vi "SortArrayData.vi"(4 "Stacked Data":i16[][][][](array[numeric]), 6 "Atts":dbl[][](array[numeric])) -> (0 "Syth App Data":i16[][][](array[numeric]), 1 "Number of Planes":i32, 2 "Att (dB)":sgl[](array[numeric]))   [LabVIEW 2022 SP3]
panel:
  in  "Case Constant\n(See Context Help)":bool=TRUE
  out "size(s) 2":i32[](array[numeric])
  out "size(s)":i32[](array[numeric])
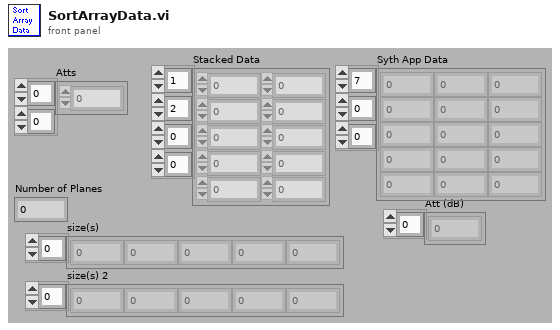
[diagram p1: front panel]
types:
  T1 = cluster{"[0]":i32, "[1]":i32, "[2]":i32, "[3]":i32}
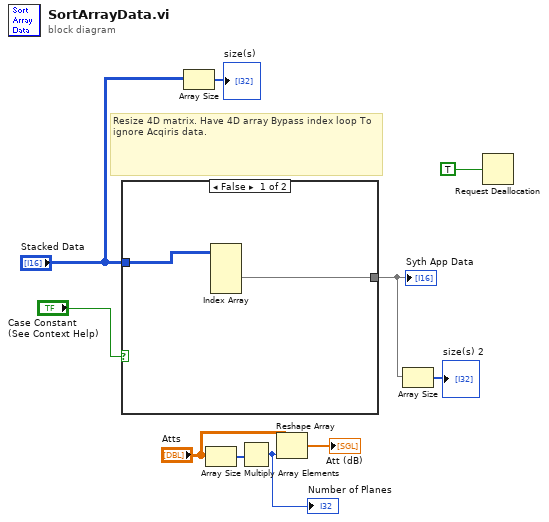
[diagram p0: block diagram]
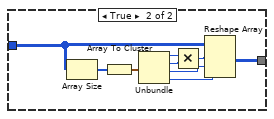
[diagram p2: hidden frame]
diagram:
  # "Resize 4D matrix. Have 4D array Bypass index loop To ignore Acqiris data."
  n1 = case shown="False" "Case Constant\n(See Context Help)" {
    tunnel: "Stacked Data" -> [w11 w13]
    tunnel: [w12 w14] -> w5
    frame False {
      n2 = Index Array(array=w11) -> (element=w12:i16[][][])  [unwired: 4 in]
    }
    frame True {
      n3 = Array Size(array=w13) -> (size(s)=w16:i32[])
      n4 = Array To Cluster(array=w16) -> (cluster=w17:T1)
      n5 = Unbundle(w17) -> ("[0]"=w15:i32, "[1]"=w21:i32, "[2]"=w19:i32, "[3]"=w18:i32)
      n6 = Multiply(x=w15, y=w21) -> (x*y=w20:i32)
      n7 = Reshape Array(w13, w20, w19, w18) -> (w14:i16[][][])
    }
  }
  "Syth App Data" <- w5
  n8 = Array Size(array="Stacked Data") -> (size(s)=→"size(s)":i32[])
  n9 = Array Size(array="Atts") -> (size(s)=w2:i32[])
  n10 = Multiply Array Elements(1:w2) -> (0:w1:i32)
  "Number of Planes" <- w1
  n11 = Reshape Array("Atts", w1) -> (→"Att (dB)":dbl[])
  n12 = Array Size(array=w5) -> (size(s)=→"size(s) 2":i32[])
  n13 = Request Deallocation(TRUE) -> ()
